vi "Projet.vi"() -> ()   [LabVIEW 2017]
panel:
  out "Alarme temperatutre":bool
  out "Alarme Pluie":bool
  out "Alarme Vent":bool
  out "Thermomètre":dbl(slide) scale=-20.0..50.0
  in  "Mise à zéro du niveau d'eau":bool=TRUE
  out "Boussole":i32(knob) scale=0.0..8.0
  in  "Stop !":bool
  out "Données Station Météo":T1
  # "N"
  # "N-O"
  # "N-E"
  # "O"
  # "E"
  # "S-E"
  # "S-O"
  # "S"
  # "1"
  # "La station est choisi gràce à un encodeur rotatif à 16 positions."
  # "La vitesse du vent est donné par l'anémomètre qui compte le nombre d'impulsions et converti cet valeur en vitesse."
  # "2"
  # "3"
  # "La quantité d'eau est donné par le pluviomètre qui compte une certaine quantité d'eau à chaque basculement."
  # "4"
  # "La direction est donné par une girouette qui sort une tension différente en fonction de la position."
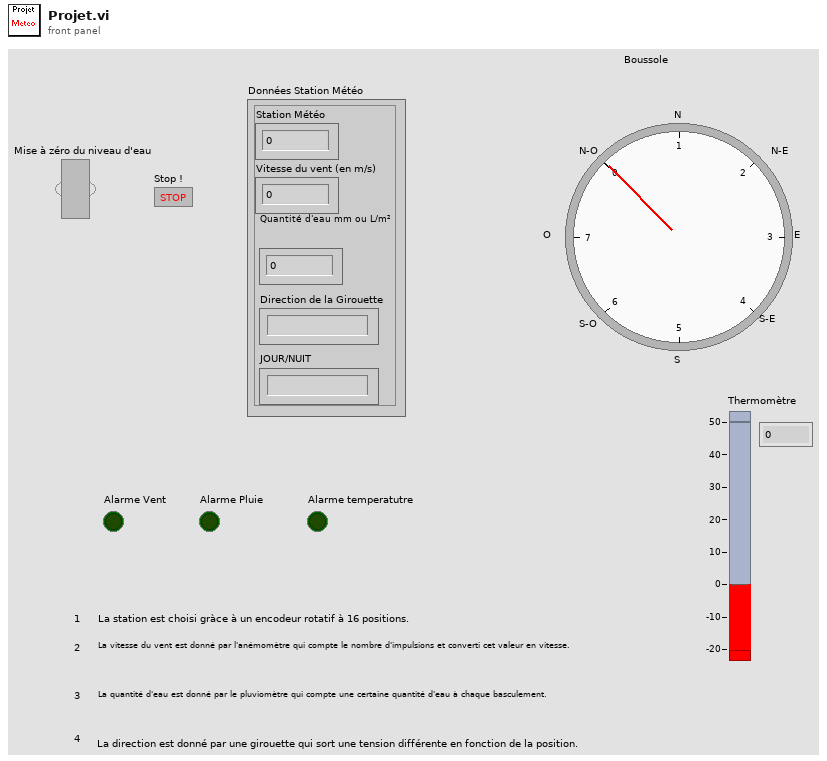
[diagram p1: front panel]
types:
  T1 = cluster{"Station Météo":i32, "Vitesse du vent (en m/s)":dbl, "Quantité d'eau mm ou L/m²":dbl, "Direction de la Girouette":string, "JOUR/NUIT":string}
  T2 = enum16{"open", "replace", "create", "open or create", "replace or create", "replace or create with confirmation"}
  T3 = cluster{"Station Météo":i32, "Vitesse (en m/s)":dbl, "Quantité de pluie (en mm)":dbl, "Direction de la Girouette":string, "JOUR/NUIT ":string}
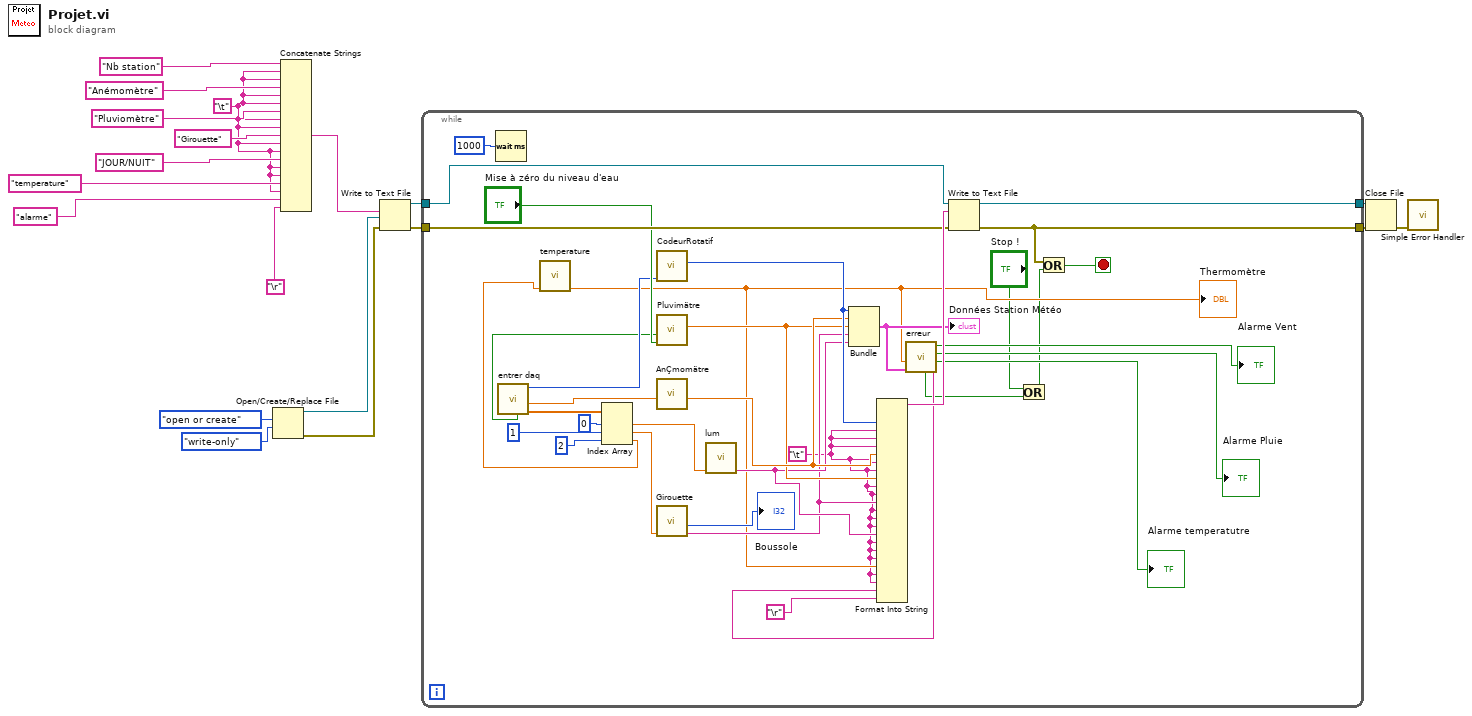
[diagram p0: block diagram]
diagram:
  w2 = "\t"
  n1 = Open/Create/Replace File(operation (0:open)=T2."open or create", access (0:read/write)=enum16{"read/write", "read-only", "write-only"}."write-only" ("accès (0 : read/write)")) -> (refnum out=w11:refnum<file>, error out=w12:errorcluster)  [unwired: 4 in, 1 out]
  n2 = Concatenate Strings("Nb station", w2, w2, "Anémomètre", w2, w2, "Pluviomètre", w2, w2, "Girouette", w2, w2, "JOUR/NUIT", w2, w2, "temperature", w2, "alarme", "\r") -> (w9:string)
  n3 = Write to Text File(file (use dialog)=w11, text=w9, error in=w12) -> (refnum out=w14:refnum<file>, error out=w13:errorcluster)  [unwired: 1 in, 1 out]
  n4 = while {
    tunnel: [w54] -> w18
    tunnel: w13 -> [w52]
    tunnel: [w49] -> w17
    tunnel: w14 -> [w50]
    stop <- w48 stop-if-true
    w25 = "\t"
    n5 = Wait (ms)(milliseconds to wait=u32 1000 ("attente (ms)")) -> ()  [unwired: 1 out]
    n6 = call "entrer daq.vi"() -> ("Tableau"=w41:dbl[], "vent"=w42:dbl, "codeur"=w44:i32, "pluie"=w43:bool)  [unwired: 8 in]
    n7 = Index Array(array=w41, index #1=0 ("indice"), index #2=1 ("indice"), index #3=2 ("indice")) -> (element #1=w37:dbl, element #2=w38:dbl, element #3=w35:dbl)
    n8 = call "temperature.vi"("Numérique"=w35) -> ("Thermomètre"=w26:dbl)  [unwired: 10 in]
    "Thermomètre" <- w26
    n9 = call "CodeurRotatif.vi"("codeur"=w44) -> ("Station Météo"=w51:i32)  [unwired: 10 in]
    n10 = call "Pluvimätre.vi"("Mise à zéro du niveau d'eau"="Mise à zéro du niveau d'eau", "data"=w43) -> ("Quantité de pluie (en mm)"=w30:dbl)  [unwired: 9 in]
    n11 = call "AnÇmomätre.vi"("vents"=w42) -> ("Vitesse (en m/s)"=w31:dbl)  [unwired: 9 in, 1 out]
    n12 = call "Girouette.vi"("girouette"=w38) -> ("Direction de la Girouette"=w27:string, "Boussole"=→"Boussole":i32)  [unwired: 9 in]
    n13 = call "lum.vi"("lum"=w37) -> ("JOUR/NUIT"=w28:string)  [unwired: 10 in]
    n14 = Bundle("Station Météo"=w51, "Vitesse (en m/s)"=w31, "Quantité de pluie (en mm)"=w30, "Direction de la Girouette"=w27, "JOUR/NUIT"=w28) -> (w45:T3)  [unwired: 1 in]
    "Données Station Météo" <- w45
    n15 = call "erreur.vi"("Données Station Météo"=w45, "Thermomètre"=w26) -> ("alarme"=w24:string, "Alarme temperatutre"=→"Alarme temperatutre":bool, "Alarme Pluie"=→"Alarme Pluie":bool, "Alarme Vent"=→"Alarme Vent":bool, "arret alarme"=w21:bool)  [unwired: 5 in]
    n16 = Format Into String(w51, w25, w25, w25, w31, w25, w25, w30, w25, w25, w27, w25, w25, w25, w28, w25, w25, w25, w26, w25, w25, w24, "\r") -> (resulting string=w53:string)  [unwired: 3 in, 1 out]
    n17 = Write to Text File(file (use dialog)=w50, text=w53, error in=w52) -> (refnum out=w49:refnum<file>, error out=w54:errorcluster)  [unwired: 1 in, 1 out]
    n18 = Or(x="Stop !", y=w21) -> (x .or. y?=w20:bool)
    n19 = Or(x=w54, y=w20) -> (x .or. y?=w48:bool)
  }
  n20 = Close File(refnum=w17, error in=w18) -> (error out=w19:errorcluster)  [unwired: 1 out]
  n21 = call <vilib>:"Simple Error Handler.vi"("error in (no error)"=w19) -> ()  [unwired: 4 in, 5 out]
